vi "GetNodeName.vi"(0 "reference in":refnum<class "ClassNode.lvclass">, 5 "error in (no error)":errorcluster) -> (14 "reference out":refnum<class "ClassNode.lvclass">, 15 "String":string, 19 "error out":errorcluster)   [LabVIEW 2012, in "ClassNode.lvclass"]
uses:
  <resource>/Framework/Providers/Open_GDS/UML/ClassNode_class/ClassNode.lvclass
  <resource>/Framework/Providers/Open_GDS/UML/MultiLineString_class/MultiLineString.lvclass
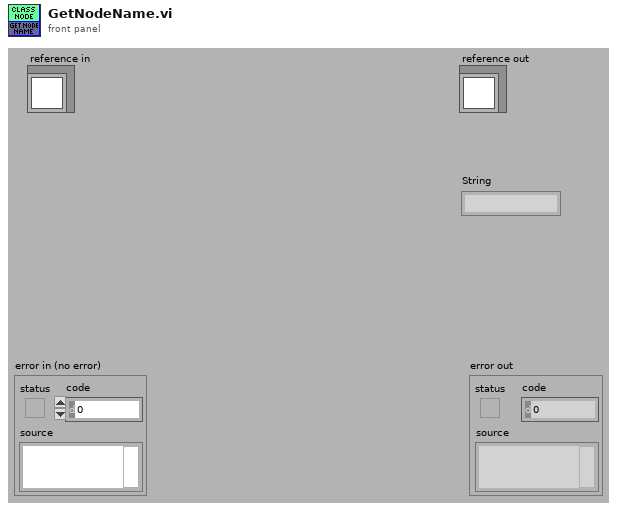
[diagram p1: front panel]
types:
  T1 = typedef "ClassNode.lvclass/ObjectAttributes.ctl" = cluster{"Base class":T2, "midHeight":dbl, "botHeight":dbl, "name":refnum<class "MultiLineString.lvclass">, "attributes":refnum<class "MultiLineString.lvclass">, "methods":refnum<class "MultiLineString.lvclass">, "DEFAULT_COMPARTMENT_HEIGHT":i32, "DEFAULT_WIDTH":i32, "DEFAULT_HEIGHT":i32, "showMethods":bool, "showAttributes":bool, "ClassPath":path}
  T2 = typedef "RectangularNode.lvclass/ObjectAttributes.ctl" = cluster{"Base class":T3, "bounds":T4}
  T3 = typedef "AbstractNode.lvclass/ObjectAttributes.ctl" = cluster{"parent":refnum<class "AbstractNode.lvclass">, "children":refnum<class "AbstractNode.lvclass">[], "Hidden":bool}
  T4 = typedef "Rectangle Rectangle2D.ctl" = cluster{"x":dbl, "y":dbl, "width":dbl, "height":dbl}
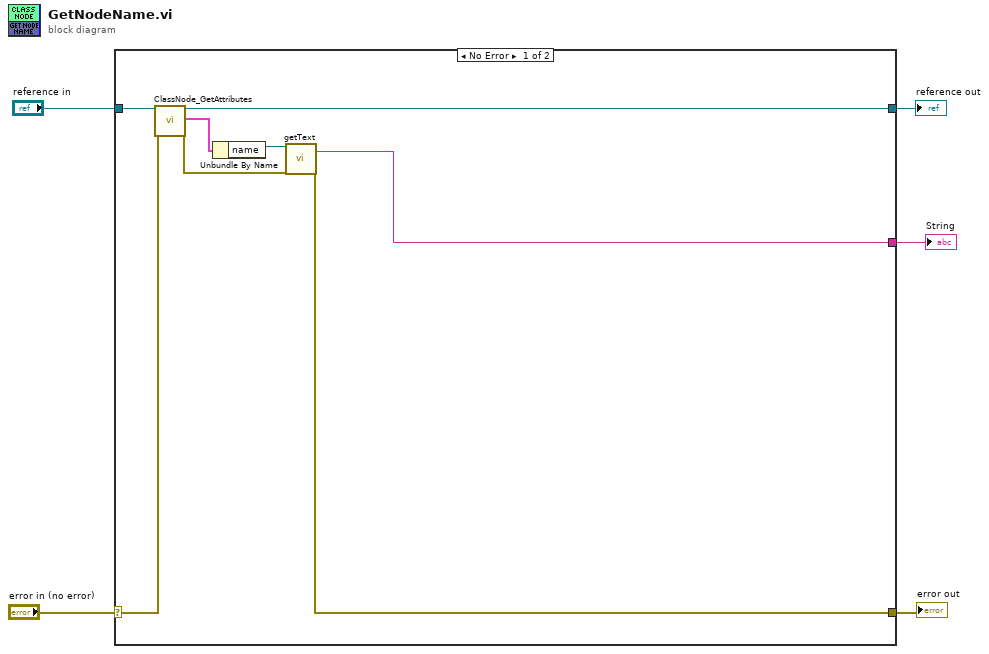
[diagram p0: block diagram]
diagram:
  n1 = case shown="No Error" "error in (no error)" {
    selector: "error in (no error)" -> [w13 w15]
    tunnel: [w7 w15] -> w4
    tunnel: [w10 w14] -> w2
    tunnel: "reference in" -> [w11 w14]
    tunnel: [w6 _] -> w1
    frame No Error {
      n2 = call <resource>:"ClassNode_GetAttributes.vi"("reference in"=w11, "error in (no error)"=w13) -> ("reference out"=w10:refnum<class "ClassNode.lvclass">, "Attributes"=w12:T1, "error out"=w8:errorcluster)  [unwired: 14 in, 1 out]
      n3 = Unbundle By Name(w12) -> ("name"=w9:refnum<class "MultiLineString.lvclass">)
      n4 = call-dynamic "getText.vi"("reference"=w9, "error in (no error)"=w8) -> ("text"=w6:string, "error out"=w7:errorcluster)  [unwired: 15 in, 1 out]
    }
    frame Error {
    }
  }
  "error out" <- w4
  "reference out" <- w2
  "String" <- w1
